vi "GetFileDependencies.vi"(9 "Overwrite LabVIEW Folder(If empty use this version of LabVIEW)":path, 11 "All Files in Dir":path[](array[path])) -> (2 "LibraryDependency":map{path, T3}(c390), 3 "FileDependency out":map{path, T1}(c390))   [LabVIEW 2020, in "DependencyChecker.lvlib"]
uses:
  DependencyChecker.lvlib
  LibraryDependentInfo.vi
  <vilib>/Utility/lvfile.llb/FT_FileTypes.ctl
  FileDependencyType.ctl
  <vilib>/Utility/lvfile.llb/NI_FileType.lvlib
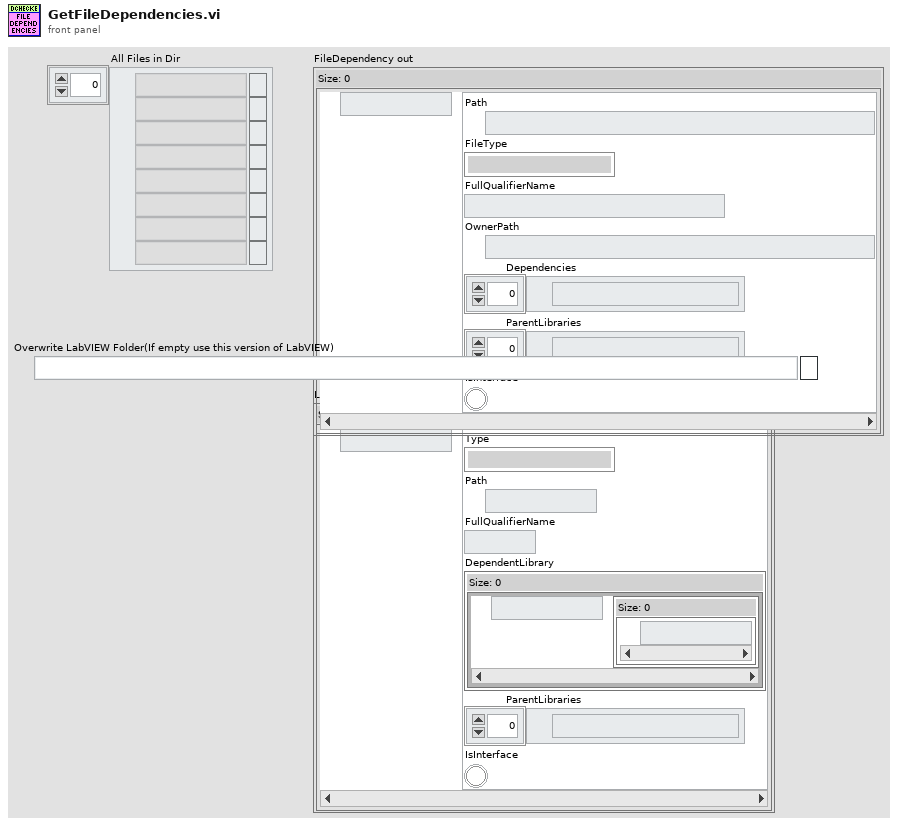
[diagram p1: front panel]
types:
  T1 = typedef "DependencyChecker.lvlib/FileDependencyType.ctl" = cluster{"Path":path, "FileType":T2, "FullQualifierName":string, "OwnerPath":path, "Dependencies":path[], "ParentLibraries":path[], "IsInterface":bool}
  T2 = typedef "NI_FileType.lvlib/FT_FileTypes.ctl" = enum32{"Invalid file/path", "Unknown type", "Instrument", "Control", "Polymorphic VI", "Project", "Library", "LVClass", "XControl", "XNode", "CIN", "Run-time menu", "Palette menu", "LLB", "Shortcut", "Directory", "Class Private Data Control", "Statechart", "MathScript .m file", "Ladder Diagram", "LVLibp"}
  T3 = typedef "DependencyChecker.lvlib/LibraryDependentInfo.vi" = cluster{"Type":T2, "Path":path, "FullQualifierName":string, "DependentLibrary":map{path, set{path}}, "ParentLibraries":path[], "IsInterface":bool}
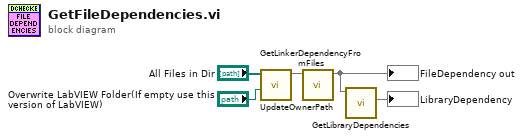
[diagram p0: block diagram]
diagram:
  n1 = call "GetLinkerDependencyFromFiles.vi"("Overwrite LabVIEW Folder(If empty use this version of LabVIEW)"="Overwrite LabVIEW Folder(If empty use this version of LabVIEW)", "All Files in Dir"="All Files in Dir") -> ("FileDependency"=w3:map{path, T1})  [unwired: 9 in]
  n2 = call "UpdateOwnerPath.vi"("FileDependency in"=w3) -> ("FileDependency out"=w4:map{path, T1})  [unwired: 10 in]
  "FileDependency out" <- w4
  n3 = call "GetLibraryDependencies.vi"("FileDependency"=w4) -> ("LibraryDependency"=→"LibraryDependency":map{path, T3})  [unwired: 10 in]
